vi "sub_Check_Rx_Packet_Validity_FSK.vi"(8 "Packet Parameters":T3, 9 "Input Bit Stream":cluster{"bit stream ":i8[][], "Enable?":bool}, 10 "FSK Init Parameters":T1) -> (1 "Output Bit Stream":T2)   [LabVIEW 2015]
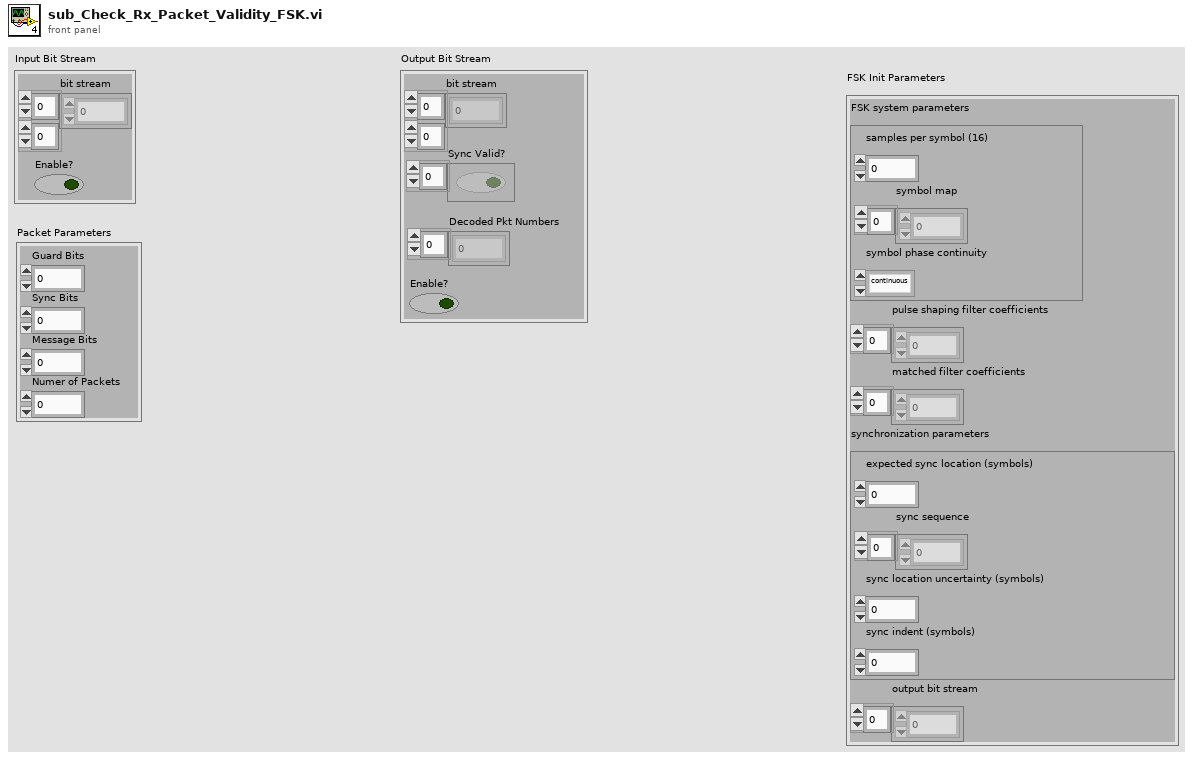
[diagram p1: front panel]
types:
  T1 = cluster{"FSK system parameters":cluster{"samples per symbol (16)":i32, "symbol map":dbl[], "symbol phase continuity":enum16{"continuous", "discontinuous"}}, "pulse shaping filter coefficients":dbl[], "matched filter coefficients":dbl[], "synchronization parameters":cluster{"expected sync location (symbols)":i32, "sync sequence":cdb[], "sync location uncertainty (symbols)":i32, "sync indent (symbols)":i32}, "output bit stream":i8[]}
  T2 = cluster{"bit stream ":i8[][], "Sync Valid?":bool[], "Decoded Pkt Numbers":u32[], "Enable?":bool}
  T3 = cluster{"Guard Bits ":i32, "Sync Bits":i32, "Message Bits":i32, "Numer of Packets":i32}
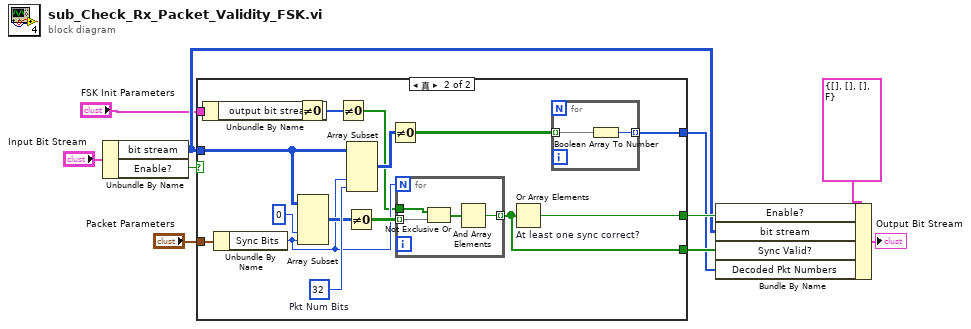
[diagram p0: block diagram]
diagram:
  n1 = Unbundle By Name("Input Bit Stream") -> ("bit stream"=w6:i8[][], "Enable?"=w9:bool)
  n2 = case shown="真" w9 {
    selector: w9 -> [w11 _]
    tunnel: w6 -> [_ w21]
    tunnel: "Packet Parameters" -> [_ w26]
    tunnel: "FSK Init Parameters" -> [_ w15]
    tunnel: [_ w20] -> w5
    tunnel: [_ w22] -> w4
    tunnel: [w11 w19] -> w7
    frame False {
    }
    frame True {
      w24 = 32  # Pkt Num Bits
      n3 = Unbundle By Name(w15) -> ("output bit stream"=w13:i8[])
      n4 = Unbundle By Name(w26) -> ("Sync Bits"=w14:i32)
      n5 = Not Equal To 0?(x=w13) -> ()  [unwired: 1 out]
      n6 = Array Subset(array=w21, index (col)=0 ("index"), length (col)=w14) -> (w17:i8[][])  [unwired: 2 in]
      n7 = Not Equal To 0?(x=w13) -> (x != 0?=w12:bool[])
      n8 = Not Equal To 0?(x=w17) -> (x != 0?=w16:bool[][])
      n9 = Array Subset(array=w21, index (col)=w14, length (col)=w24) -> (w23:i8[][])  [unwired: 2 in]
      n10 = Not Equal To 0?(x=w23) -> (x != 0?=w18:bool[][])
      n11 = for {
        N: w14 -> [_]
        tunnel: [w30] -> w20 mode=indexing
        tunnel: w12 -> [w28]
        tunnel: w16 -> [w27] mode=indexing
        n12 = Not Exclusive Or(1:w27, 2:w28) -> (0:w29:bool[])
        n13 = And Array Elements(Boolean array=w29) -> (logical AND=w30:bool)
      }
      n14 = Or Array Elements "At least one sync correct?"(Boolean array=w20) -> (logical OR=w19:bool)
      n15 = for {
        tunnel: [w32] -> w22 mode=indexing
        tunnel: w18 -> [w31] mode=indexing
        n16 = Boolean Array To Number(Boolean array=w31) -> (number=w32:u32)
      }
    }
  }
  n17 = Bundle By Name(cluster=T2 {"bit stream "=[], "Sync Valid?"=[], "Decoded Pkt Numbers"=[], "Enable?"=FALSE} ("Output Bit Stream"), "Enable?"=w7, "bit stream"=w6, "Sync Valid?"=w5, "Decoded Pkt Numbers"=w4) -> (→"Output Bit Stream":T2)
